vi "Pause.vi"(8 "error in (no error)":errorcluster, 11 "Pause user event":refnum<user-event>) -> (0 "error out":errorcluster, 3 "user event Out":refnum<user-event>)   [LabVIEW 2011]
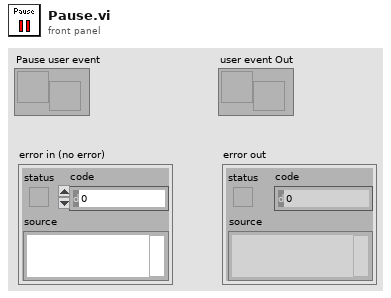
[diagram p1: front panel]
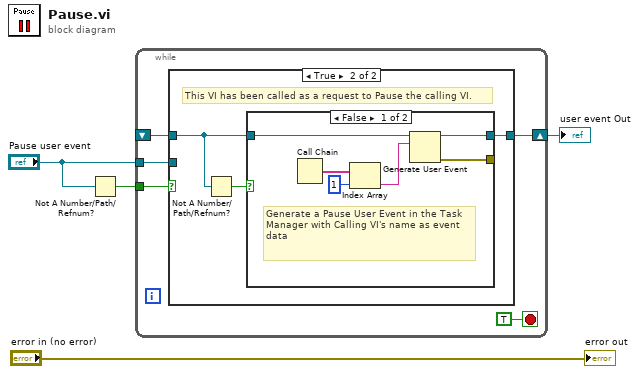
[diagram p0: block diagram]
diagram:
  n1 = Not A Number/Path/Refnum?(number/path/refnum="Pause user event") -> (NaN/Path/Refnum?=w4:bool)
  n2 = while {
    tunnel: w4 -> [w9]
    shift-right: [w8] -> w2
    shift-left: _ -> [w5]
    tunnel: "Pause user event" -> [w7]
    stop <- TRUE stop-if-true
    n3 = case shown="True" w9 {
      tunnel: [w10 w13] -> w8
      tunnel: w7 -> [w10 _]
      tunnel: w5 -> [_ w11]
      frame False {
        # "This VI has been called to stored a ref\nto a new user event."
      }
      frame True {
        # "This VI has been called as a request to Pause the calling VI."
        n4 = Not A Number/Path/Refnum?(number/path/refnum=w11) -> (NaN/Path/Refnum?=w12:bool)
        n5 = case shown="False" w12 {
          tunnel: w11 -> [w19 w20]
          tunnel: [w18 w20] -> w13
          tunnel: [w14 _] -> _
          frame False {
            # "Generate a Pause User Event in the Task Manager with Calling VI's name as event data"
            n6 = Call Chain() -> (call chain=w17:string[])
            n7 = Index Array(array=w17, index=1) -> (element=w15:string)
            n8 = Generate User Event(user event=w19, event data cluster=w15) -> (user event out=w18:refnum<user-event>, error out=w14:errorcluster)  [unwired: 1 in]
          }
          frame True {
            # "Task Manager is not open to handle\nthis request."
          }
        }
      }
    }
  }
  "user event Out" <- w2
  "error out" <- "error in (no error)"
